vi "a_n__v1.vi"(11 "ƒÁ[n-1]":ext) -> (3 "a[n]":ext)   [LabVIEW 2020]
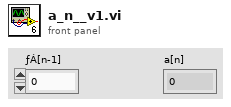
[diagram p1: front panel]
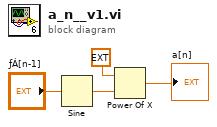
[diagram p0: block diagram]
diagram:
  n1 = Sine(x="ƒÁ[n-1]") -> (sin(x)=w3:ext)
  n2 = Power Of X(1:w3, 2:ext -2.0) -> (0:→"a[n]":ext)
